vi "Read Size.vi"(8 "error in (no error)":errorcluster, 11 "file in":refnum<class "node.lvclass">) -> (0 "error out":errorcluster, 2 "Size":i64, 3 "file out":refnum<class "node.lvclass">)   [LabVIEW 2021, in "d7.lvlib" / "node.lvclass"]
uses:
  node.lvclass
  node.lvclass/node.ctl
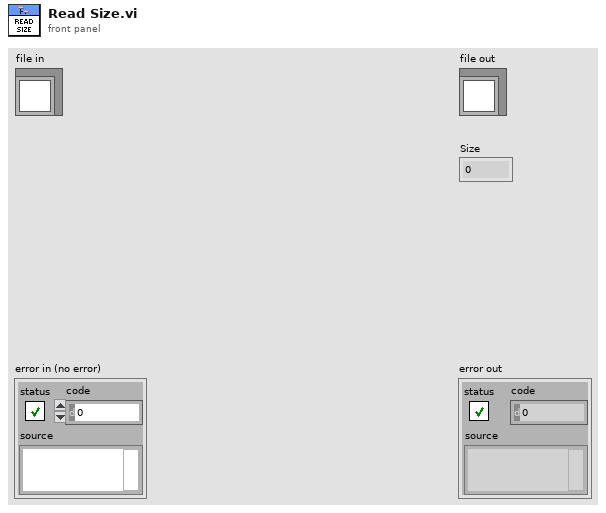
[diagram p1: front panel]
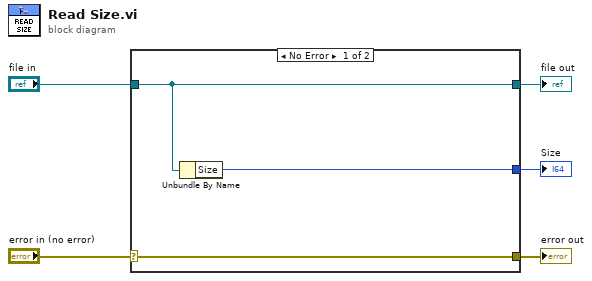
[diagram p0: block diagram]
diagram:
  n1 = case shown="No Error" "error in (no error)" {
    selector: "error in (no error)" -> [w8 w9]
    tunnel: [w8 w9] -> w4
    tunnel: [w7 w10] -> w2
    tunnel: "file in" -> [w7 w10]
    tunnel: [w6 _] -> w1
    frame No Error {
      n2 = Unbundle By Name(w7) -> ("Size"=w6:i64)
    }
    frame Error {
    }
  }
  "error out" <- w4
  "file out" <- w2
  "Size" <- w1
